vi "Channel Measurement Limit Set All.vi"(0 "instrument handle":refnum<k15>, 2 "Measurement":string, 5 "LimitTypeVal":i32[](array[numeric])=[0], 6 "error in (no error)":errorcluster {"code" format="%.0x"}, 8 "EndYVal":dbl[](array[numeric])=[1.0] format="%.2p", 11 "BeginXVal":dbl[](array[numeric])=[0.0] format="%.2p", 13 "EndXVal":dbl[](array[numeric])=[1.0] format="%.2p", 17 "BeginYVal":dbl[](array[numeric])=[0.0] format="%.2p") -> (20 "instrument handle out":refnum<k15>, 26 "error out":errorcluster {"code" format="%.0x"})   [LabVIEW 2014, in "Agilent NA.lvlib"]
doc: "Sets all data for limit segments."
uses:
  Agilent NA.lvlib
  AgNA.dll
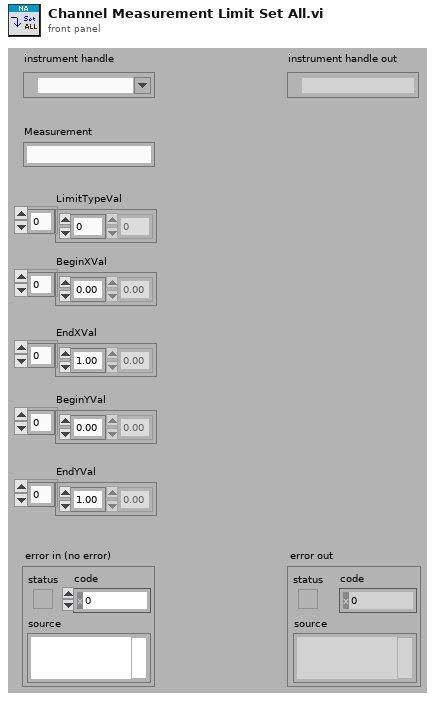
[diagram p1: front panel]
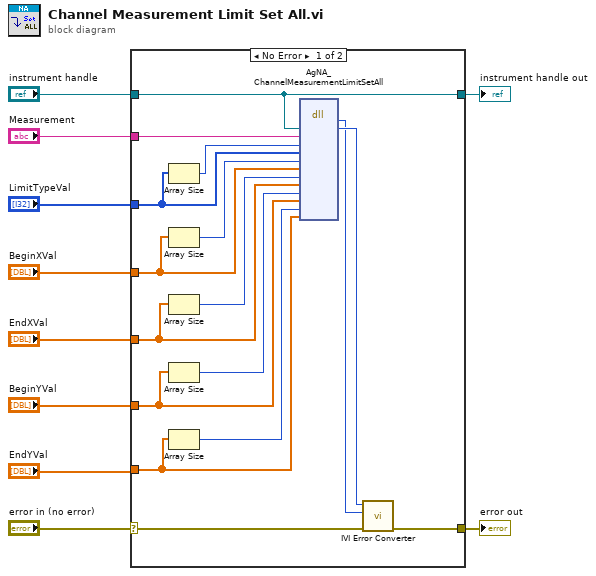
[diagram p0: block diagram]
diagram:
  n1 = case shown="No Error" "error in (no error)" {
    selector: "error in (no error)" -> [w24 w28]
    tunnel: [w23 w28] -> w10
    tunnel: "Measurement" -> [w22 _]
    tunnel: "LimitTypeVal" -> [w11 _]
    tunnel: "BeginXVal" -> [w19 _]
    tunnel: "EndXVal" -> [w17 _]
    tunnel: "BeginYVal" -> [w15 _]
    tunnel: "EndYVal" -> [w13 _]
    tunnel: [w21 w27] -> w2
    tunnel: "instrument handle" -> [w21 w27]
    frame No Error {
      n2 = Array Size(array=w11) -> (size(s)=w12:i32)
      n3 = Array Size(array=w19) -> (size(s)=w20:i32)
      n4 = Array Size(array=w17) -> (size(s)=w18:i32)
      n5 = Array Size(array=w15) -> (size(s)=w16:i32)
      n6 = Array Size(array=w13) -> (size(s)=w14:i32)
      n7 = dll-call lib="AgNA**.dll" fn="AgNA_ChannelMeasurementLimitSetAll"("Vi"=w21, "Measurement"=w22, "LimitTypeValBufferSize"=w12, "LimitTypeVal"=w11, "BeginXValBufferSize"=w20, "BeginXVal"=w19, "EndXValBufferSize"=w18, "EndXVal"=w17, "BeginYValBufferSize"=w16, "BeginYVal"=w15, "EndYValBufferSize"=w14, "EndYVal"=w13) -> (w25:i32, "Vi"=w26:u32)  [unwired: 14 in, 2 out]
      n8 = call "IVI Error Converter.vi"("error in (no error)"=w24, "IVI error code (0)"=w25, "instrument handle"=w26) -> ("error out"=w23:errorcluster)  [unwired: 7 in, 1 out]
    }
    frame Error {
    }
  }
  "error out" <- w10
  "instrument handle out" <- w2
